vi "Set servo angle.vi"(11 "Target Index":dbl) -> ()   [LabVIEW 2011]
uses:
  Robot Global Data.vi
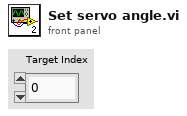
[diagram p1: front panel]
types:
  T1 = cluster{"Position":cluster{"X":dbl, "Y":dbl}, "Distance (ft)":dbl}[]
  T2 = cluster{"Position":cluster{"X":dbl, "Y":dbl}, "Distance (ft)":dbl}
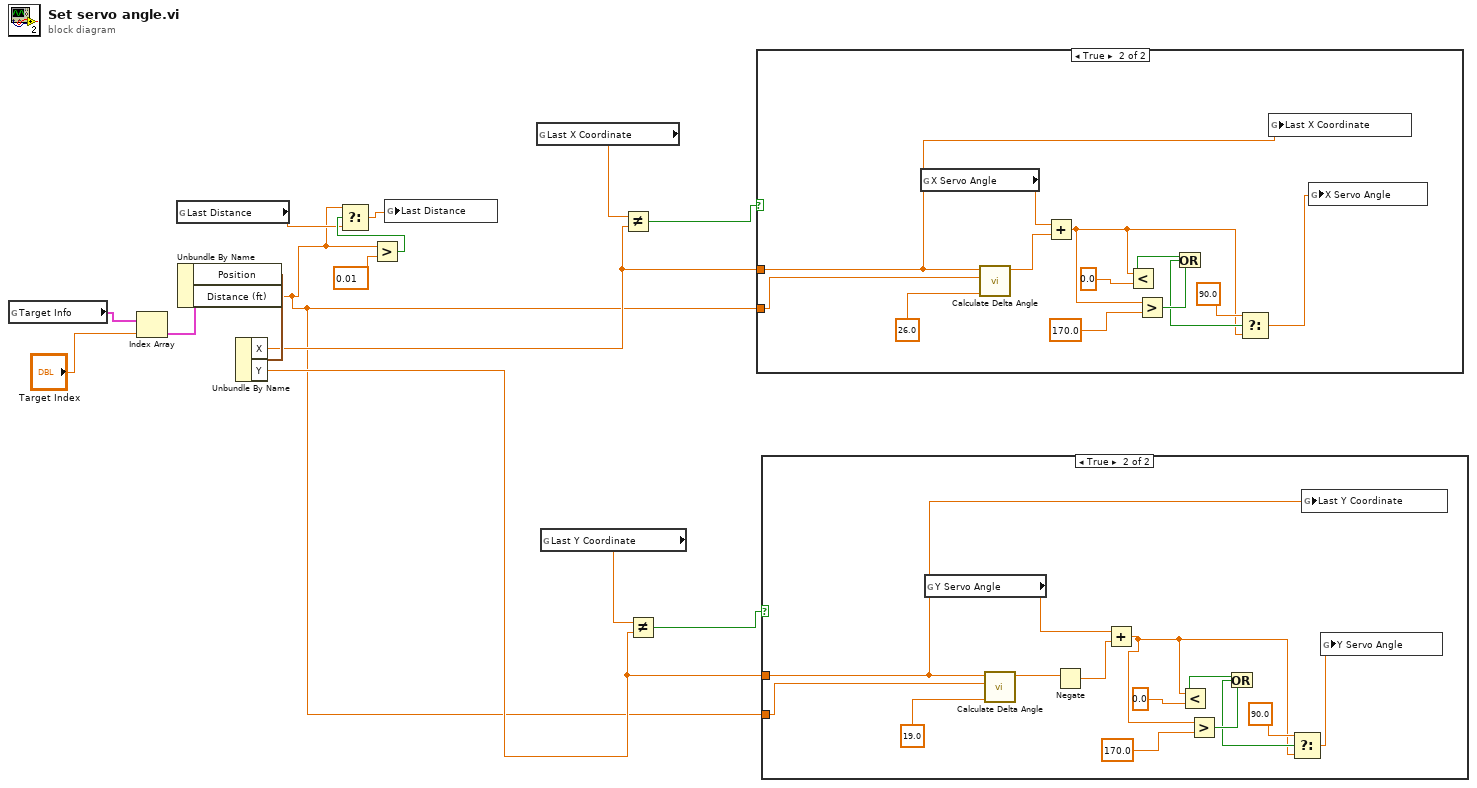
[diagram p0: block diagram]
diagram:
  n1 = global read "Robot Global Data.vi" "Target Info"() -> (w15:T1)
  n2 = Index Array(array=w15, index="Target Index") -> (element=w14:T2)
  n3 = global read "Robot Global Data.vi" "Last Distance"() -> (w7:dbl)
  n4 = Unbundle By Name(w14) -> ("Position"=w13:cluster{"X":dbl, "Y":dbl}, "Distance (ft)"=w6:dbl)
  n5 = Unbundle By Name(w13) -> ("X"=w12:dbl, "Y"=w11:dbl)
  n6 = Greater?(x=w6, y=0.01) -> (0:w8:bool)
  n7 = Select(t=w6, s=w8, f=w7) -> (s? t:f=w5:dbl)
  n8 = global write "Robot Global Data.vi" "Last Distance"(w5) -> ()
  n9 = global read "Robot Global Data.vi" "Last X Coordinate"() -> (w1:dbl)
  n10 = global read "Robot Global Data.vi" "Last Y Coordinate"() -> (w3:dbl)
  n11 = Not Equal?(x=w1, y=w12) -> (x != y?=w2:bool)
  n12 = Not Equal?(x=w3, y=w11) -> (x != y?=w4:bool)
  n13 = case shown="True" w2 {
    tunnel: w12 -> [_ w24]
    tunnel: w6 -> [_ w25]
    frame False {
    }
    frame True {
      n14 = global read "Robot Global Data.vi" "X Servo Angle"() -> (w26:dbl)
      n15 = call "Calculate Delta Angle.vi"("Degrees 0-1"=26.0, "Distance (ft)"=w25, "X"=w24) -> ("Output Angle Delta"=w27:dbl)  [unwired: 8 in]
      n16 = Add(x=w26, y=w27) -> (x+y=w16:dbl)
      n17 = Less?(x=w16, y=0.0) -> (x < y?=w21:bool)
      n18 = Greater?(x=w16, y=170.0) -> (0:w20:bool)
      n19 = Or(x=w21, y=w20) -> (x .or. y?=w19:bool)
      n20 = Select(t=90.0, s=w19, f=w16) -> (s? t:f=w17:dbl)
      n21 = global write "Robot Global Data.vi" "Last X Coordinate"(w24) -> ()
      n22 = global write "Robot Global Data.vi" "X Servo Angle"(w17) -> ()
    }
  }
  n23 = case shown="True" w4 {
    tunnel: w11 -> [_ w37]
    tunnel: w6 -> [_ w40]
    frame False {
    }
    frame True {
      n24 = global read "Robot Global Data.vi" "Y Servo Angle"() -> (w41:dbl)
      n25 = call "Calculate Delta Angle.vi"("Degrees 0-1"=19.0, "Distance (ft)"=w40, "X"=w37) -> ("Output Angle Delta"=w39:dbl)  [unwired: 8 in]
      n26 = Negate(x=w39) -> (-x=w38:dbl)
      n27 = Add(x=w41, y=w38) -> (x+y=w30:dbl)
      n28 = Less?(x=w30, y=0.0) -> (x < y?=w34:bool)
      n29 = Greater?(x=w30, y=170.0) -> (0:w33:bool)
      n30 = Or(x=w34, y=w33) -> (x .or. y?=w32:bool)
      n31 = Select(t=90.0, s=w32, f=w30) -> (s? t:f=w29:dbl)
      n32 = global write "Robot Global Data.vi" "Last Y Coordinate"(w37) -> ()
      n33 = global write "Robot Global Data.vi" "Y Servo Angle"(w29) -> ()
    }
  }
